vi "Handle Error.vi"(8 "error in (no error)":errorcluster, 11 "IObserver in":refnum<class "IObserver.lvclass">) -> (0 "error out":errorcluster, 2 "stop actor?":bool=TRUE, 3 "IObserver out":refnum<class "IObserver.lvclass">)   [LabVIEW 2015, in "IObserver.lvlib" / "IObserver.lvclass"]
doc: "(<B>Filename</B>: Actor Framework.lvlib:Actor.lvclass:Handle Error.vi)\n\nDefines how the actor handles an error that occurred while processing a message. By default, this method does nothing except stop the actor."
uses:
  IObserver.lvclass
  <vilib>/ActorFramework/Actor/Actor.lvclass
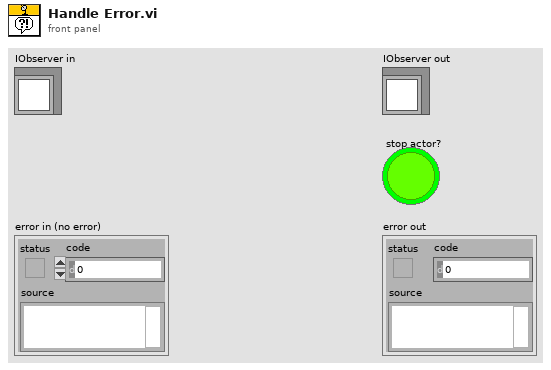
[diagram p1: front panel]
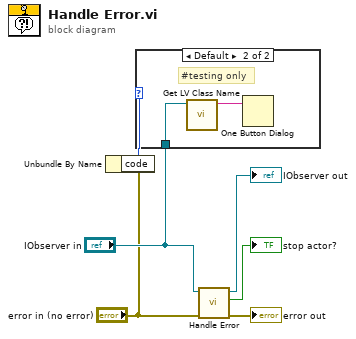
[diagram p0: block diagram]
diagram:
  n1 = Unbundle By Name("error in (no error)") -> ("code"=w1:i32)
  n2 = case shown="Default" w1 {
    tunnel: "IObserver in" -> [_ w8]
    frame 43 {
    }
    frame Default {
      # "#testing only"
      n3 = call <vilib>:"Get LV Class Name.vi"("object"=w8) -> ("class name"=w7:string)  [unwired: 9 in, 1 out]
      n4 = One Button Dialog(message=w7) -> ()  [unwired: 1 in, 1 out]
    }
  }
  n5 = call-parent "Handle Error.vi"("error in (no error)"="error in (no error)", "Actor in"="IObserver in") -> ("error out"=→"error out":errorcluster, "stop actor?"=→"stop actor?":bool, "Actor out"=→"IObserver out":refnum<class "IObserver.lvclass">)  [unwired: 7 in]
